vi "Detect.vi"(6 "VI to busy":refnum<vi>, 8 "error in (no error)":errorcluster, 10 "Targets in":T7 {"Filtered Targets"."IP Mode" items=["Static"=1, "DHCP/Link-Local"=2, "Link-Local Only"=4, "DHCP Only"=8]}, 11 "Ctl Refs in":T1) -> (0 "error out":errorcluster, 1 "Execution State":T10, 2 "Targets out":T7 {"Filtered Targets"."IP Mode" items=["Static"=1, "DHCP/Link-Local"=2, "Link-Local Only"=4, "DHCP Only"=8]}, 3 "Ctl Refs out":T1)   [LabVIEW 2013]
uses:
  Controls/Refs.ctl
  Controls/Button Refs.ctl
  Controls/Tab Ctl Refs.ctl
  types/TabStateType.ctl
  Controls/Indicator Refs.ctl
  Controls/Slider Refs.ctl
  Controls/Control Refs.ctl
  Controls/Targets.ctl
  Controls/Detected.ctl
  types/MAX Sys Cfg Target Information.ctl
  types/ExecutionStateType.ctl
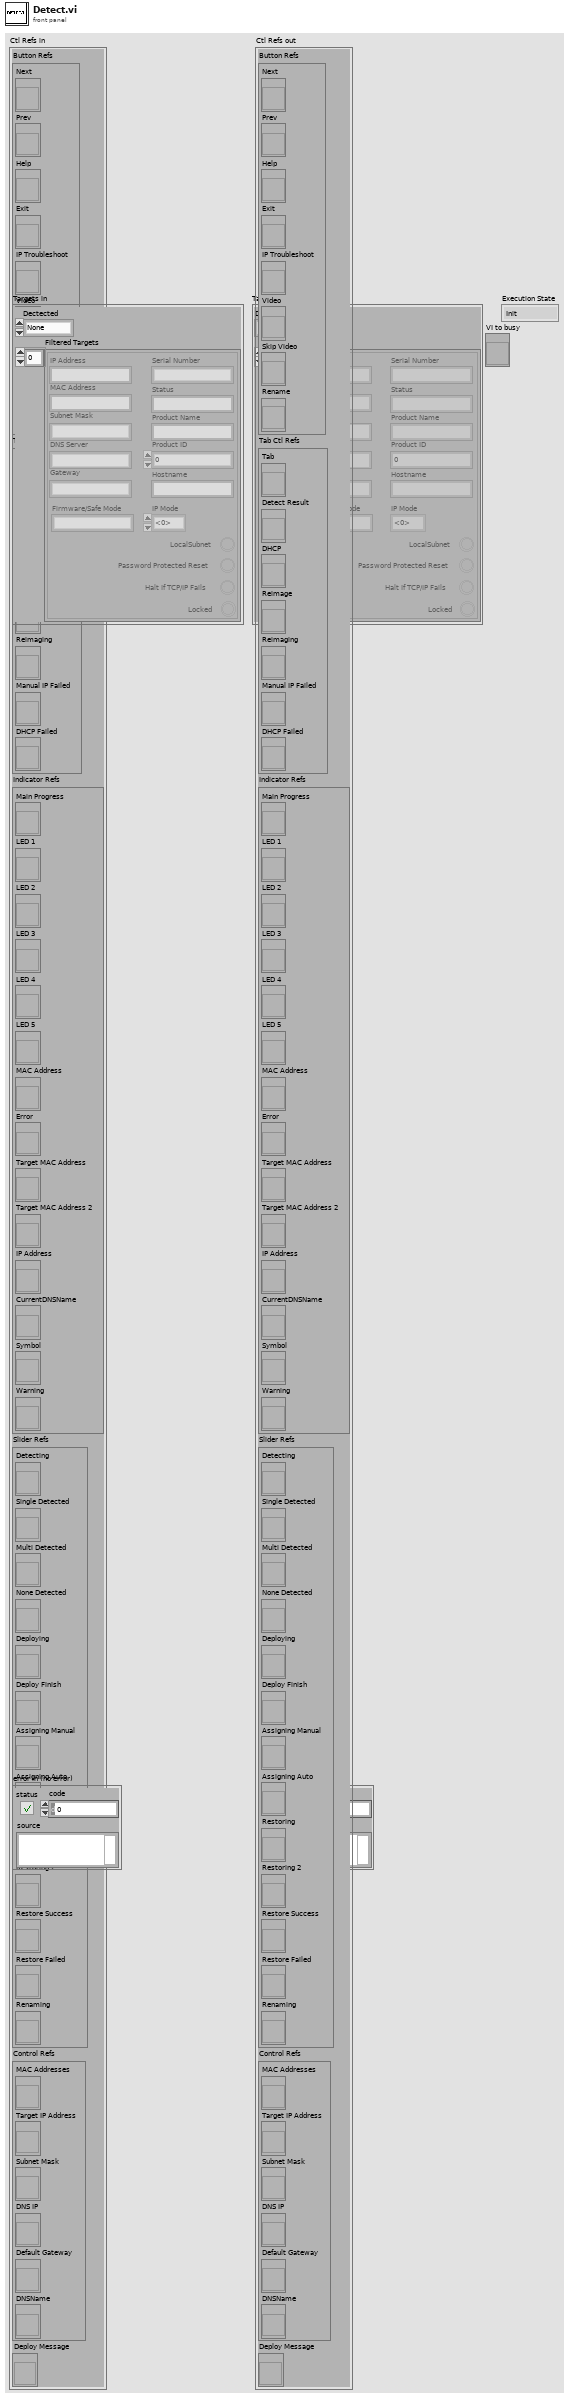
[diagram p1: front panel]
types:
  T1 = typedef "Refs.ctl" = cluster{"Button Refs":T2, "Tab Ctl Refs":T3, "Indicator Refs":T4, "Slider Refs":T5, "Control Refs":T6, "Deploy Message":refnum<vi>}
  T2 = typedef "Button Refs.ctl" = cluster{"Next":refnum<vi>, "Prev":refnum<vi>, "Help":refnum<vi>, "Exit":refnum<vi>, "IP Troubleshoot":refnum<vi>, "Video":refnum<vi>, "Skip Video":refnum<vi>, "Rename":refnum<vi>}
  T3 = typedef "Tab Ctl Refs.ctl" = cluster{"Tab":refnum<vi>, "Detect Result":refnum<vi>, "DHCP":refnum<vi>, "Reimage":refnum<vi>, "Reimaging":refnum<vi>, "Manual IP Failed":refnum<vi>, "DHCP Failed":refnum<vi>}
  T4 = typedef "Indicator Refs.ctl" = cluster{"Main Progress":refnum<vi>, "LED 1":refnum<vi>, "LED 2":refnum<vi>, "LED 3":refnum<vi>, "LED 4":refnum<vi>, "LED 5":refnum<vi>, "MAC Address":refnum<vi>, "Error":refnum<vi>, "Target MAC Address":refnum<vi>, "Target MAC Address 2":refnum<vi>, "IP Address":refnum<vi>, "CurrentDNSName":refnum<vi>, "Symbol":refnum<vi>, "Warning":refnum<vi>}
  T5 = typedef "Slider Refs.ctl" = cluster{"Detecting":refnum<vi>, "Single Detected":refnum<vi>, "Multi Detected":refnum<vi>, "None Detected":refnum<vi>, "Deploying":refnum<vi>, "Deploy Finish":refnum<vi>, "Assigning Manual":refnum<vi>, "Assigning Auto":refnum<vi>, "Restoring":refnum<vi>, "Restoring 2":refnum<vi>, "Restore Success":refnum<vi>, "Restore Failed":refnum<vi>, "Renaming":refnum<vi>}
  T6 = typedef "Control Refs.ctl" = cluster{"MAC Addresses":refnum<vi>, "Target IP Address":refnum<vi>, "Subnet Mask":refnum<vi>, "DNS IP":refnum<vi>, "Default Gateway":refnum<vi>, "DNSName":refnum<vi>}
  T7 = typedef "Targets.ctl" = cluster{"Dectected":T8, "Filtered Targets":T9[]}
  T8 = typedef "Detected.ctl" = enum16{"None", "Failed", "Single", "Multi"}
  T9 = typedef "MAX Sys Cfg Target Information.ctl" = cluster{"MAC Address":string, "IP Address":string, "Status":string, "Product Name":string, "Hostname":string, "Firmware/Safe Mode":string, "Subnet Mask":string, "Gateway":string, "DNS Server":string, "Serial Number":string, "Product ID":u32, "Locked ":bool, "LocalSubnet":bool, "Halt If TCP/IP Fails":bool, "Password Protected Reset":bool, "IP Mode":i32}
  T10 = typedef "ExecutionStateType.ctl" = enum16{"Init", "Welcome", "Idle", "Detect", "Run Detection", "Detect Fail", "Detect One", "Detect Mult", "Deploy", "DHCP", "Static IP", "Run Deployment", "Connect Verify", "Exit", "Video Wait", "Success", "Troubleshoot", "Troubleshoot 2", "RenameDNS"}
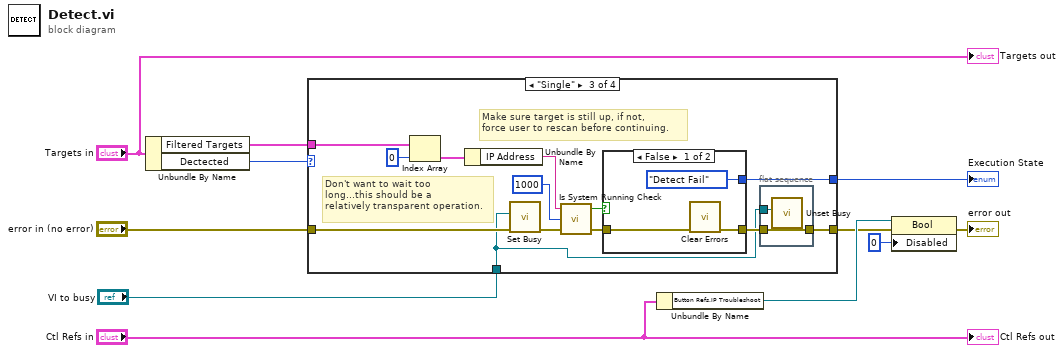
[diagram p0: block diagram]
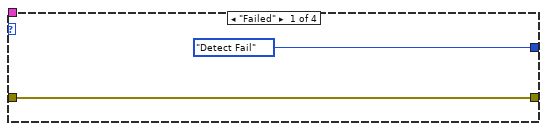
[diagram p2: hidden frame]
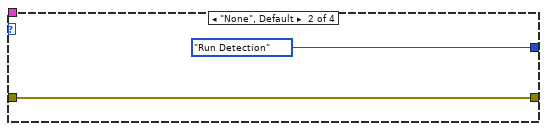
[diagram p3: hidden frame]
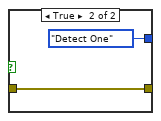
[diagram p4: hidden frame]
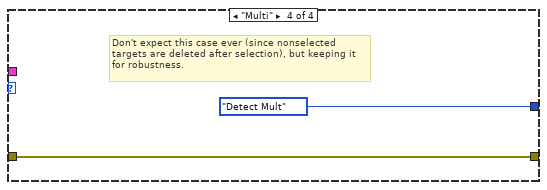
[diagram p5: hidden frame]
diagram:
  n1 = Unbundle By Name("Targets in") -> ("Filtered Targets"=w4:T9[], "Dectected"=w10:T8)
  n2 = case shown="\"Single\"" w10 {
    tunnel: [ExecutionStateType."Detect Fail" ("Enum") ExecutionStateType."Run Detection" ("Enum") w26 ExecutionStateType."Detect Mult" ("Enum")] -> w5
    tunnel: "error in (no error)" -> [w12 w14 w25 w36]
    tunnel: [w12 w14 w18 w36] -> w8
    tunnel: w4 -> [_ _ w20 _]
    tunnel: "VI to busy" -> [_ _ w16 _]
    frame "Failed" {
    }
    frame "None", Default {
    }
    frame "Single" {
      # "Don't want to wait too\nlong...this should be a\nrelatively transparent operation."
      # "Make sure target is still up, if not, \nforce user to rescan before continuing."
      n3 = Index Array(array=w20, index=0) -> (element=w27:T9)
      n4 = Unbundle By Name(w27) -> ("IP Address"=w22:string)
      n5 = call <vilib>:"Set Busy.vi"("error in (no error)"=w25, "VI reference (current VI)"=w16) -> ("error out"=w19:errorcluster)  [unwired: 8 in, 1 out]
      n6 = call "Is System Running Check.vi"("error in (no error)"=w19, "connect timeout in ms (4s)"=u32 1000 ("timeout ms (10000)"), "IP Address"=w22) -> ("error out"=w24:errorcluster, "x = y?"=w21:bool)  [unwired: 1 in]
      n7 = case shown="False" w21 {
        tunnel: [ExecutionStateType."Detect Fail" ("Enum") ExecutionStateType."Detect One" ("Enum")] -> w26
        tunnel: w24 -> [w32 w34]
        tunnel: [w31 w34] -> w17
        frame False {
          n8 = call <vilib>:"Clear Errors.vi"("error in (no error)"=w32) -> ("error out"=w31:errorcluster)  [unwired: 6 out]
        }
        frame True {
        }
      }
      n9 = flat-sequence {
        tunnel: [w30] -> w18
        tunnel: w17 -> [w30]
        tunnel: w16 -> [w29]
        frame #0 {
          n10 = call <vilib>:"Unset Busy.vi"("VI reference (current VI)"=w29) -> ()  [unwired: 10 in, 1 out]
        }
      }
    }
    frame "Multi" {
      # "Don't expect this case ever (since nonselected\ntargets are deleted after selection), but keeping it\nfor robustness."
    }
  }
  "Execution State" <- w5
  n11 = Unbundle By Name("Ctl Refs in") -> ("Button Refs.IP Troubleshoot"=w11:refnum<vi>)
  n12 = property on="Property Node" class="Bool"(reference=w11, error in=w8, "Disabled"=u8 0) -> (error out=→"error out":errorcluster)  [unwired: 1 out]
  "Targets out" <- "Targets in"
  "Ctl Refs out" <- "Ctl Refs in"
